vi "SS2 Live_First Image.vi"() -> (0 "error out":errorcluster, 3 "Image":T1(plugin-control))   [LabVIEW 2019]
panel:
  in  "# Iterations":i32 format="%.0p"
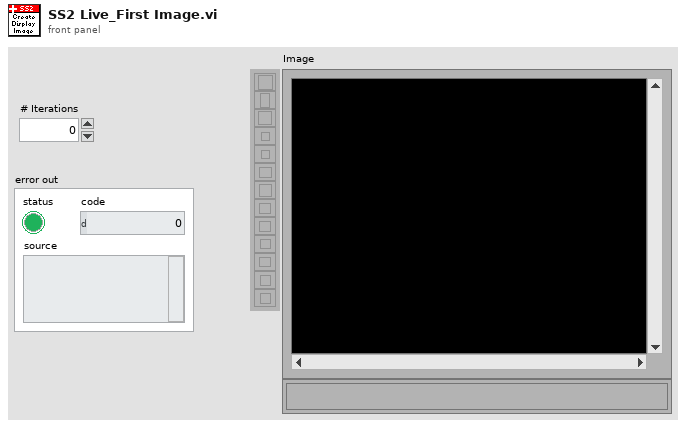
[diagram p1: front panel]
types:
  T1 = typedef "IMAQ Image.ctl" = refnum<image>
  T2 = typedef "Image Type" = u32
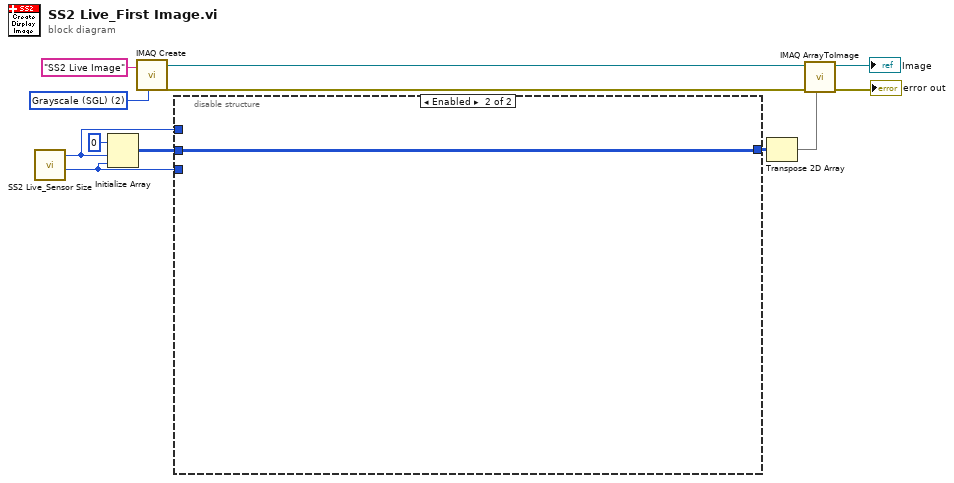
[diagram p0: block diagram]
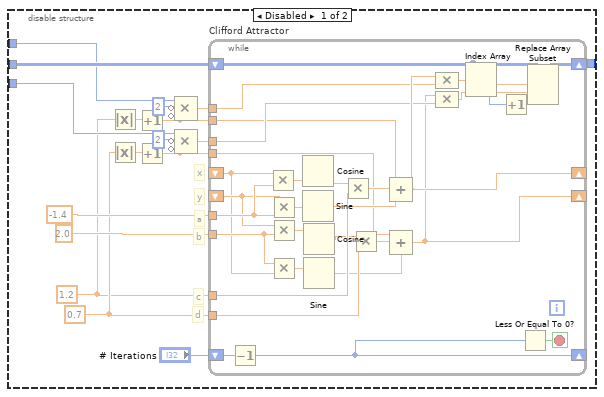
[diagram p2: hidden frame]
diagram:
  w12 = T2 2 items=["Grayscale (U8)", "Grayscale (I16)", "Grayscale (SGL)", "Complex (CSG)", "RGB (U32)", "HSL (U32)", "RGB (U64)", "Grayscale (U16)"] ("Image Type")
  n1 = call "SS2 Live_Sensor Size.vi"() -> ("Y size"=w1:i32, "X size"=w2:i32)  [unwired: 10 in]
  n2 = Initialize Array(u16 0 ("element"), w2, w1) -> (w9:u16[][])
  n3 = call "IMAQ Create"("Image Name"="SS2 Live Image", "Image Type"=w12) -> ("New Image"=w4:T1, "error out"=w3:errorcluster)  [unwired: 3 in]
  n4 = disable-structure shown="Enabled" {
    disable-tunnel: w9 -> [w29 w61]
    disable-tunnel: [w28 w61] -> w8
    disable-tunnel: w2 -> [w25 _]
    disable-tunnel: w1 -> [w20 _]
    frame Disabled {
      w14 = 0.7
      w13 = 1.2
      # "d"
      # "c"
      # "b"
      # "a"
      # "y"
      # "x"
      n5 = Absolute Value(x=w13) -> (abs(x)=w26:dbl)
      n6 = Absolute Value(x=w14) -> (abs(x)=w21:dbl)
      n7 = Increment(x=w26) -> (x+1=w18:dbl)
      n8 = Increment(x=w21) -> (x+1=w17:dbl)
      n9 = Compound Arithmetic op=MULTIPLY(w25, invert 2 ("value"), invert w18) -> (w23:dbl)
      n10 = Compound Arithmetic op=MULTIPLY(w20, invert 2 ("value"), invert w17) -> (w19:dbl)
      n11 = while "Clifford Attractor" {
        shift-right: [w44] -> _
        shift-left: _ -> [w35]
        shift-right: [w37] -> _
        shift-left: _ -> [w36]
        tunnel: -1.4 ("Numeric") -> [w60]
        tunnel: 2.0 ("Numeric") -> [w52]
        tunnel: w13 -> [w57]
        tunnel: w14 -> [w49]
        shift-right: [w30] -> w28
        shift-left: w29 -> [w34]
        shift-right: [w31] -> _
        shift-left: "# Iterations" -> [w43]
        tunnel: w23 -> [w41]
        tunnel: w19 -> [w40]
        tunnel: w18 -> [w39]
        tunnel: w17 -> [w38]
        stop <- w42 stop-if-true
        n12 = Decrement(x=w43) -> (x-1=w31:i32)
        n13 = Multiply(x=w35, y=w60) -> (x*y=w59:dbl)
        n14 = Multiply(x=w36, y=w60) -> (x*y=w56:dbl)
        n15 = Multiply(x=w36, y=w52) -> (x*y=w53:dbl)
        n16 = Multiply(x=w52, y=w35) -> (x*y=w51:dbl)
        n17 = Cosine(x=w59) -> (cos(x)=w58:dbl)
        n18 = Sine(x=w56) -> (sin(x)=w55:dbl)
        n19 = Cosine(x=w53) -> (cos(x)=w50:dbl)
        n20 = Sine(x=w51) -> (sin(x)=w47:dbl)
        n21 = Multiply(x=w58, y=w57) -> (x*y=w54:dbl)
        n22 = Multiply(x=w50, y=w49) -> (x*y=w48:dbl)
        n23 = Compound Arithmetic op=ADD(w39, w54, w55) -> (w44:dbl)
        n24 = Compound Arithmetic op=ADD(w38, w48, w47) -> (w37:dbl)
        n25 = Compound Arithmetic op=MULTIPLY(w44, w41) -> (w33:dbl)
        n26 = Compound Arithmetic op=MULTIPLY(w37, w40) -> (w32:dbl)
        n27 = Index Array(array=w34, index (row)=w33, index (col)=w32) -> (element=w45:u16)
        n28 = Increment(x=w45) -> (x+1=w46:u16)
        n29 = Less Or Equal To 0?(x=w31) -> (x <= 0?=w42:bool)
        n30 = Replace Array Subset(array=w34, new element=w46, index (row)=w33, index (col)=w32) -> (w30:u16[][])
      }
    }
    frame Enabled {
    }
  }
  n31 = Transpose 2D Array(2D array=w8) -> (transposed array=w6:u16[][])
  n32 = call "IMAQ ArrayToImage"("Image Pixels (Float)"=w6, "error in (no error)"=w3, "Image"=w4) -> ("error out"=→"error out":errorcluster, "Image Out"=→"Image":T1)  [unwired: 7 in]
